vi "GPIB_RQS_W_StopGen.vi"(8 "error in":errorcluster caption="entrée d'erreur", 9 "StopRef":refnum<vi>, 10 "timeout ms (488.2 global)":i32, 11 "address string":string) -> (0 "error out":errorcluster caption="sortie d'erreur", 1 "Stopped":bool, 2 "poll response byte":i16)   [LabVIEW 2019]
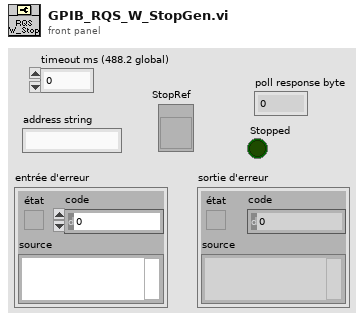
[diagram p1: front panel]
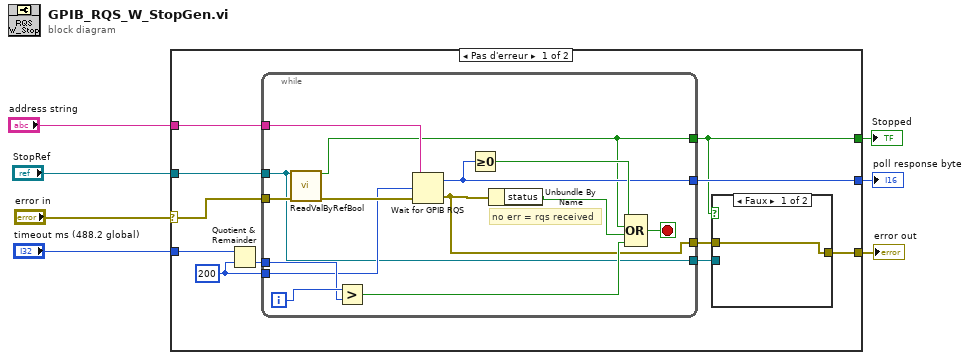
[diagram p0: block diagram]
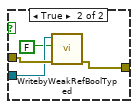
[diagram p2: hidden frame]
diagram:
  n1 = case shown="Pas d'erreur" "error in" {
    selector: "error in" -> [w12 w38]
    tunnel: "StopRef" -> [w18 _]
    tunnel: "timeout ms (488.2 global)" -> [w17 _]
    tunnel: "address string" -> [w14 _]
    tunnel: [w11 w38] -> w4
    tunnel: [w13 _] -> w3
    tunnel: [w8 _] -> w1
    frame No Error {
      w16 = u32 200 ("milliseconds to wait")
      n2 = Quotient & Remainder(x=w17, y=w16) -> (floor(x/y)=w15:u32)  [unwired: 1 out]
      n3 = while {
        tunnel: w18 -> [w24]
        tunnel: w12 -> [w37]
        tunnel: w16 -> [w28]
        tunnel: w15 -> [w35]
        tunnel: w14 -> [w33]
        tunnel: [w27] -> w13
        tunnel: [w26] -> w8
        tunnel: [w25] -> w10
        tunnel: [w24] -> w9
        i -> [w36]
        stop <- w34 stop-if-true
        # "no err = rqs received"
        n4 = call <userlib>:"ReadValByRefBool.vi"("Control Ref"=w24, "error in"=w37) -> ("Valeur"=w26:bool, "error out"=w30:errorcluster)  [unwired: 12 in]
        n5 = Greater?(x=w36, y=w35) -> (0:w31:bool)
        n6 = Wait for GPIB RQS(2:w30, 3:w28, 4:w33) -> (0:w25:errorcluster, 1:w27:i16)
        n7 = Greater Or Equal To 0?(x=w27) -> (x >= 0?=w29:bool)
        n8 = Unbundle By Name(w25) -> ("status"=w32:bool)
        n9 = Compound Arithmetic op=OR(w29, w26, w32, w31) -> (w34:bool)
      }
      n10 = case shown="Faux" w8 {
        tunnel: [w19 w23] -> w11
        tunnel: w10 -> [w19 w22]
        tunnel: w9 -> [_ w21]
        frame False {
        }
        frame True {
          n11 = call <userlib>:"WritebyWeakRefBoolTyped.vi"("error in"=w22, "Valeur"=FALSE ("t"), "Control Ref"=w21) -> ("error out"=w23:errorcluster)  [unwired: 8 in]
        }
      }
    }
    frame Error {
    }
  }
  "error out" <- w4
  "poll response byte" <- w3
  "Stopped" <- w1
